vi "9214_Initialize_From9213.vi"(7 "Module Model":T1=enum."NI 9205", 8 "error in (no error)":errorcluster, 9 "Slot Settings":T2, 11 "9213 in":refnum<class "9213.lvclass">) -> (0 "error out":errorcluster, 3 "9214 out":refnum<class "9214.lvclass">)   [LabVIEW 2015, in "Modules.lvlib" / "9214.lvclass"]
uses:
  9214.lvclass
  RSI Module/Slot Settings.ctl
  9213/9213.lvclass
  RSI Module/Module Models.ctl
  RSI Module/RSI Module.lvclass
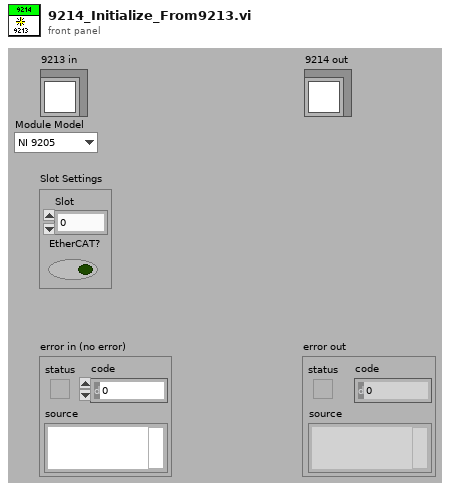
[diagram p1: front panel]
types:
  T1 = typedef "Modules.lvlib/RSI Module.lvclass/Module Models.ctl" = enum16{"Empty", "NI 9201", "NI 9203", "NI 9205", "NI 9206", "NI 9207", "NI 9208", "NI 9211", "NI 9213", "NI 9214", "NI 9215", "NI 9217", "NI 9219", "NI 9221", "NI 9225", "NI 9227", "NI 9229", "NI 9233", "NI 9234", "NI 9235", "NI 9236", "NI 9237", "NI 9239", "NI 9263", "NI 9264", "NI 9265", "NI 9269", "NI 9375", "NI 9401", "NI 9402", "NI 9403", "NI 9411", "NI 9421", "NI 9422", "NI 9423", "NI 9425", "NI 9426", "NI 9435", "NI 9472", "NI 9474", "NI 9475", "NI 9476", "NI 9477", "NI 9478", "NI 9481", "NI 9482", "NI 9485"}
  T2 = typedef "Modules.lvlib/RSI Module.lvclass/Slot Settings.ctl" = cluster{"Slot":u32, "EtherCAT?":bool}
  T3 = typedef "Modules.lvlib/9213.lvclass/Conversion Time.ctl" = u16
  T4 = typedef "Modules.lvlib/9213.lvclass/Thermocouple Type.ctl" = u8
  T5 = typedef "Modules.lvlib/9213.lvclass/Measurement Units.ctl" = u8
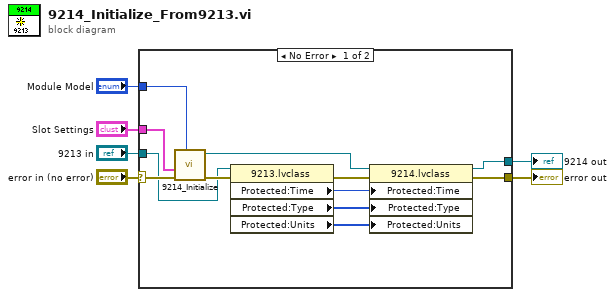
[diagram p0: block diagram]
diagram:
  n1 = case shown="No Error" "error in (no error)" {
    selector: "error in (no error)" -> [w18 w19]
    tunnel: [w7 w19] -> w5
    tunnel: [w8 _] -> w1
    tunnel: "9213 in" -> [w12 _]
    tunnel: "Slot Settings" -> [w17 _]
    tunnel: "Module Model" -> [w16 _]
    frame No Error {
      n2 = call "9214_Initialize.vi"("Module Model"=w16, "error in (no error)"=w18, "Slot Settings"=w17) -> ("error out"=w14:errorcluster, "9214 out"=w15:refnum<class "9214.lvclass">)  [unwired: 7 in]
      n3 = property class="9213.lvclass"(reference=w12, error in=w14) -> (error out=w13:errorcluster, "Protected:Time"=w11:T3, "Protected:Type"=w10:T4[], "Protected:Units"=w9:T5[])  [unwired: 1 out]
      n4 = property class="9214.lvclass"(reference=w15, error in=w13, "Protected:Time"=w11, "Protected:Type"=w10, "Protected:Units"=w9) -> (reference out=w8:refnum<class "9214.lvclass">, error out=w7:errorcluster)
    }
    frame Error {
    }
  }
  "error out" <- w5
  "9214 out" <- w1
